vi "Handle Exit.vi"(8 "error in":errorcluster, 9 "Stop Argument":T1, 10 "Admin in":refnum<class "Delacor_lib_QMH_Module Admin.lvclass">, 11 "VI reference":refnum<vi>) -> (0 "error out":errorcluster, 3 "Wait for Module to stop?":bool)   [LabVIEW 2025, in "Acquisition.lvlib"]
doc: "This VI handles the Exit Message for a DQMH Singleton module. \n\nThis VI determines if the message was received via the Stop Request or not. If the Exit message was received via the Request Event to Stop the module then there is no need to send the Stop Request again. If it was not, then the Stop Request needs to be fired so the Event Handling Loop can stop.\n\nThis VI also hides the Main.vi Front Panel, this is to ensure that the module stays in memory until the very last step in the Main.vi which is to close the front panel.\n_____\nBased on DQMH Project Template 4.0.0.47.\n_____\nBased on DQMH Dev Tools: Project Template 7.1.0.1503."
uses:
  Acquisition.lvlib
  <vilib>/Delacor/Delacor QMH/Libraries/Module Admin_class/Delacor_lib_QMH_Module Admin.lvclass
  Stop Argument--cluster.ctl
  <vilib>/Delacor/Delacor QMH/Libraries/Module Admin_class/Delacor_lib_QMH_Module Admin.lvclass/Delacor_lib_QMH_Module Admin.ctl
  <vilib>/Delacor/Delacor QMH/Libraries/Module Admin_class/Delacor_lib_QMH_Get External Launch.vi
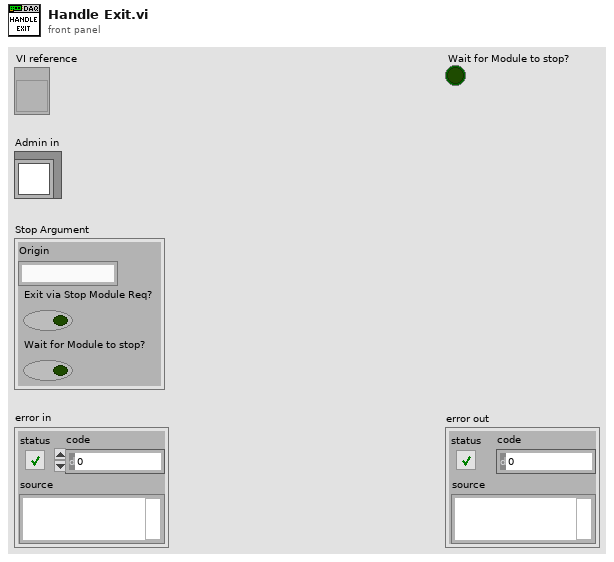
[diagram p1: front panel]
types:
  T1 = typedef "Acquisition.lvlib/Stop Argument--cluster.ctl" = cluster{"Origin":string, "Exit via Stop Module Req?":bool, "Wait for Module to stop?":bool}
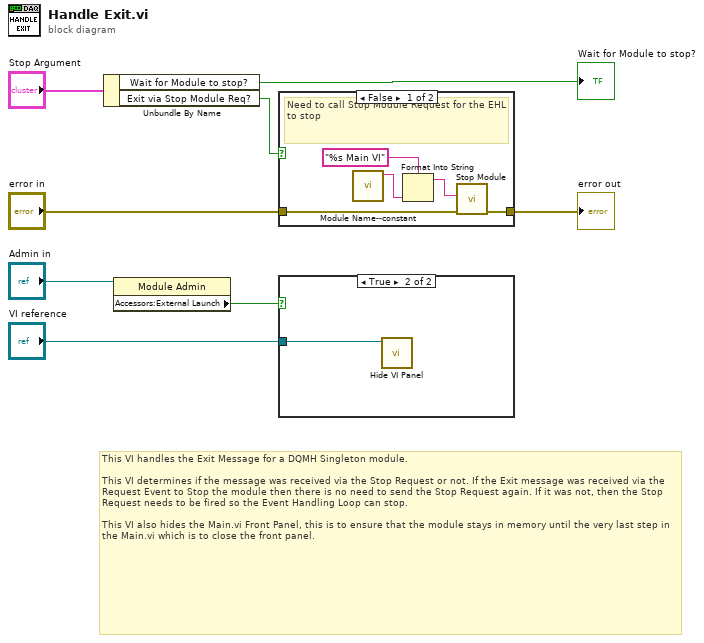
[diagram p0: block diagram]
diagram:
  # "This VI handles the Exit Message for a DQMH Singleton module. \n\nThis VI determines if the message was received via the Stop Request or not. If the Exit message was received via the Request Event to Stop the module then there is no need to send the Stop Request again. If it was not, then the Stop Request needs to be fired so the Event Handling Loop can stop.\n\nThis VI also hides the Main.vi Front Panel, this is to ensure that the module stays in memory until the very last step in the Main.vi which is to close the front panel."
  n1 = Unbundle By Name("Stop Argument") -> ("Wait for Module to stop?"=→"Wait for Module to stop?":bool, "Exit via Stop Module Req?"=w3:bool)
  n2 = property on="Property Node" class="Module Admin"(reference="Admin in") -> ("Accessors:External Launch"=w1:bool)  [unwired: 1 in, 2 out]
  n3 = case "Exit came from Stop Module Request?" shown="False" w3 {
    tunnel: [w11 w14] -> w5
    tunnel: "error in" -> [w9 w14]
    frame False {
      # "Need to call Stop Module Request for the EHL to stop"
      n4 = call "Module Name--constant.vi"() -> ("Module Name"=w10:string)  [unwired: 11 in]
      n5 = Format Into String(format string="%s Main VI", w10) -> (resulting string=w12:string)  [unwired: 2 in, 1 out]
      n6 = call "Stop Module.vi"("error in"=w9, "Origin"=w12) -> ("error out"=w11:errorcluster)  [unwired: 9 in]
    }
    frame True {
      # "no need to call Stop Module Request again."
    }
  }
  "error out" <- w5
  n7 = case shown="True" w1 {
    tunnel: "VI reference" -> [_ w15]
    frame False {
    }
    frame True {
      n8 = call "Hide VI Panel.vi"("VI"=w15) -> ()  [unwired: 10 in, 1 out]
    }
  }
